vi "Test App Removed Process Returned.vi"(8 "error in (no error)":errorcluster, 11 "Rig Test in":refnum<class "Application Dev Test.lvclass">) -> (0 "error out":errorcluster, 3 "Rig Test out":refnum<class "Application Dev Test.lvclass">)   [LabVIEW 2020, in "Application Dev Test.lvclass"]
uses:
  Application Dev Test.lvclass
  C:/Program Files (x86)/National Instruments/LabVIEW 2020/vi.lib/Astemes/LUnit/Test Case.lvclass
  source/Framework/Process/Process.lvclass
  source/Framework/Process/Process.lvclass/Process.ctl
  source/Framework/Application/Application.lvclass/Application.ctl
  <vilib>/Astemes/LUnit/Test Case.lvclass/Test Case.ctl
  <vilib>/Astemes/LUnit/LUnit Assertion Result.lvclass/LUnit Assertion Result.ctl
  <vilib>/Astemes/LUnit/LUnit Test Case Result.lvclass/LUnit Test Case Result.ctl
  <vilib>/Astemes/LUnit/LUnit Method Result.lvclass/LUnit Method Result.ctl
  ee0d5f56-39d8-4792-922a-7306bed340d5.vi
  source/Framework/Application/Private/Add Process to Map.vi
  source/Framework/Application/Private/Start Idle Processes if Running.vi
  source/Framework/Application/Private/Throw Error If Process Already in App.vi
  source/Framework/Process/Protected/Messaging/Enqueue Message.vi
  source/Framework/Process/Public/Lifecycle/Get Lifecycle State.vi
  source/Framework/Process/Protected/SubVIs/Set Context.vi
  source/Framework/Application/Private/Remove Process from App.vi
  source/Framework/Application/Private/Parse Process Name.vi
  source/Framework/Application/Private/Remove Process from Map.vi
  source/Framework/Process/Protected/SubVIs/Clear Context.vi
  <vilib>/Astemes/LUnit/Palette/Pass.vi
  <vilib>/Astemes/LUnit/Palette/Fail.vi
  <vilib>/Astemes/LUnit/Compare Variants.vi
  <vilib>/Astemes/LUnit/Describe Comparison.vi
  <vilib>/Astemes/LUnit/Set Assertion Type.vi
  source/Framework/Process/Private/SubVIs/Wait for finish.vi
  source/Framework/Process/Private/SubVIs/Set Lifecycle State.vi
  source/Framework/Application/Public/Get Process.vi
  source/Framework/Process/Private/SubVIs/Handle Debug Data.vi
  <vilib>/Utility/error.llb/Clear Errors.vi
  source/Framework/Process/Public/Lifecycle/Leave Process Loop.vi
  source/Framework/Process/Protected/Messaging/Request Message.vi
  <vilib>/AdvancedString/Delimited String to 1D String Array.vi
  <vilib>/Astemes/LUnit/Add test result.vi
  <vilib>/Astemes/LUnit/LUnit Write Passed.vi
  <vilib>/Astemes/LUnit/LUnit Write Message.vi
  <vilib>/Astemes/LUnit/LUnit Write Description.vi
  <vilib>/Astemes/LUnit/Variant to string.vi
  <vilib>/Astemes/LUnit/LUnit Write Assertion Type.vi
  source/Framework/Application/Private/Retrieve Process from App.vi
  source/Framework/Application/Private/Get Process from Map.vi
  source/Framework/Logging/Log Debug.vi
  <vilib>/AdvancedString/1D String Array to Delimited String.vi
  <vilib>/Utility/High Resolution Relative Seconds.vi
  source/Framework/Process/Private/SubVIs/Enqueue Request Message.vi
  <vilib>/Astemes/LUnit/LUnit Record Assertion Result.vi
  <vilib>/Astemes/LUnit/LUnit Aggregate Assertion Results.vi
  <vilib>/Astemes/LUnit/Assertion Result/LUnit Read Status.vi
  <vilib>/Astemes/LUnit/LUnit Read Message.vi
  <vilib>/Astemes/LUnit/LUnit Read Description.vi
  <vilib>/Astemes/LUnit/Method Result/LUnit Merge Status.vi
  <vilib>/Astemes/LUnit/LUnit Concatenate result strings.vi
  source/Framework/Application/Application.lvclass
  C:/Git/astemes-triarc-framework/source/Framework/Process/Process.lvclass
  <vilib>/Utility/error.llb/Error Cluster From Error Code.vi
  source/Framework/Process/Private/SubVIs/Wait for Response Message.vi
  <vilib>/Utility/Data Type/Get Type Information.vi
  <vilib>/Utility/LVClass/Get LV Class Name.vi
  <vilib>/Astemes/LUnit/LUnit Assertion Result.lvclass
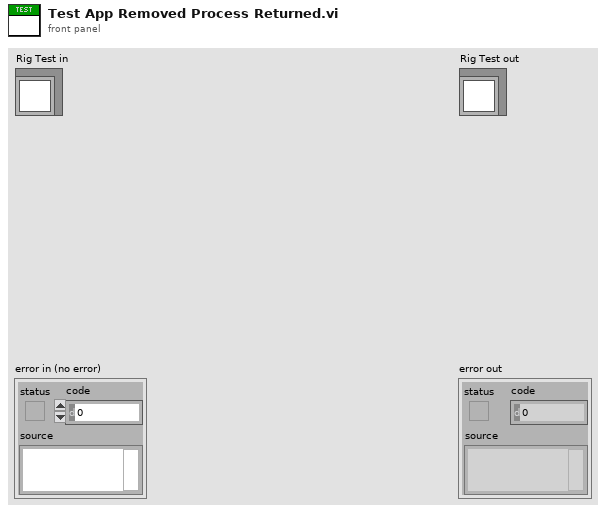
[diagram p1: front panel]
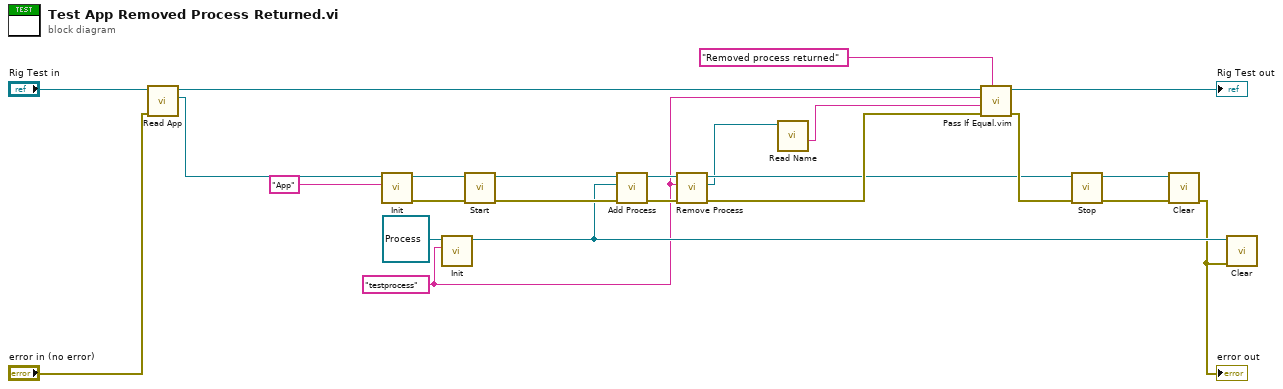
[diagram p0: block diagram]
diagram:
  w1 = "testprocess" ("Name")
  n1 = call "Read App.vi"("error in (no error)"="error in (no error)", "Application Test In"="Rig Test in") -> ("App out"=w23:refnum<class "Application.lvclass">, "Application Test Out"=w13:refnum<class "Application Dev Test.lvclass">)  [unwired: 7 in, 1 out]
  n2 = call-dynamic "Init.vi"("Name"="App", "Process In"=w23) -> ("error out"=w14:errorcluster, "Process Out"=w15:refnum<class "Application.lvclass">)  [unwired: 8 in]
  n3 = call-dynamic "Init.vi"("Name"=w1, "Process In"=refnum<class "Process.lvclass"> refnum ("Process.lvclass")) -> ("Process Out"=w5:refnum<class "Process.lvclass">)  [unwired: 8 in, 1 out]
  n4 = call "Start.vi"("error in (no error)"=w14, "Process In"=w15) -> ("error out"=w16:errorcluster, "Process Out"=w6:refnum<class "Application.lvclass">)  [unwired: 7 in, 1 out]
  n5 = call "Add Process.vi"("error in (no error)"=w16, "Process"=w5, "Application In"=w6) -> ("error out"=w20:errorcluster, "Application Out"=w8:refnum<class "Application.lvclass">)  [unwired: 7 in]
  n6 = call "Remove Process.vi"("error in (no error)"=w20, "Process Name"=w1, "Application In"=w8) -> ("error out"=w9:errorcluster, "App Process"=w3:refnum<class "Process.lvclass">, "Application Out"=w7:refnum<class "Application.lvclass">)  [unwired: 6 in]
  n7 = call "Read Name.vi"("Process In"=w3) -> ("Name"=w2:string)  [unwired: 7 in, 3 out]
  n8 = call "Pass If Equal.vim"("Description"="Removed process returned", "error in (no error)"=w9, "Actual"=w2, "Expected"=w1, "LUnit Test Case In"=w13) -> ("error out"=w18:errorcluster, "LUnit Test Case Out"=→"Rig Test out":refnum<class "Application Dev Test.lvclass">)  [unwired: 5 in]
  n9 = call "Stop.vi"("error in (no error)"=w18, "Process In"=w7) -> ("error out"=w11:errorcluster, "Process Out"=w10:refnum<class "Application.lvclass">)  [unwired: 7 in, 1 out]
  n10 = call-dynamic "Clear.vi"("error in (no error)"=w11, "Application In"=w10) -> ("error out"=w4:errorcluster)  [unwired: 9 in]
  "error out" <- w4
  n11 = call-dynamic "Clear.vi"("error in (no error)"=w4, "Process In"=w5) -> ()  [unwired: 9 in, 1 out]
